vi "FPGATest.vi"() -> ()   [LabVIEW 2016]
uses:
  <vilib>/Platform/TimedLoop/XDataNode/timing_clust.ctl
  <vilib>/Platform/TimedLoop/XDataNode/nitl_modes.ctl
  <vilib>/Platform/TimedLoop/XDataNode/wakeup.ctl
  <userlib>/_NI SPI IP/FPGA/Controllers/Public/Transfer Settings.ctl
  <userlib>/_NI SPI IP/FPGA/Controllers/Public/Slave Transfer Settings.ctl
  <vilib>/rvi/Emulation/niFpgaSctlEmulationGetInTimedLoop.vi
  <vilib>/rvi/Emulation/niFpgaEmulationReportErrorSimple.vi
  <vilib>/rvi/Emulation/niFpgaGetClockAttributes.vi
  <vilib>/rvi/Emulation/niFpgaCriticalErrorInLSC.vi
  <vilib>/rvi/eio/common/nirviEmuTemplateMethod_errors.vi
  <vilib>/platform/TimedLoop/XDataNode/XDataNode.xnode
  <vilib>/eio/EIONode/EIONode.xnode
  <userlib>/_NI SPI IP/FPGA/Controllers/NI SPI IP FPGA.lvlib
  <vilib>/Platform/TimedLoop/XDataNode/XDNodeRunTimeDep.lvlib
panel:
  out "ready for input":bool
  in  "start strobe":bool
  in  "MOSI output enable done":bool=TRUE
  out "read data":u64 format="%.0x"
  out "read data valid":bool
  in  "data to write":u64 format="%.0x"
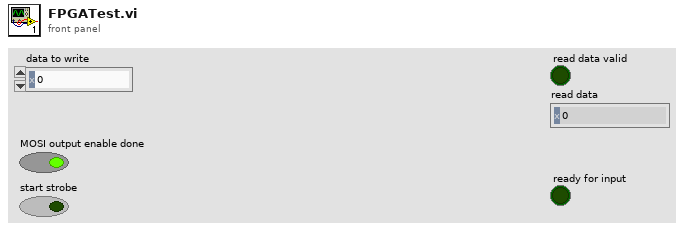
[diagram p1: front panel]
types:
  T1 = typedef "XDNodeRunTimeDep.lvlib/timing_clust.ctl" = cluster{"Expected End [f-1]":u64, "Actual End [f-1]":u64, "Finished Late? [f-1]":bool, "Expected End [i-1]":u64, "Actual End [i-1]":u64, "Finished Late? [i-1]":bool, "Expected Start [i]":u64, "Actual Start [i]":u64, "Expected Start [f]":u64, "Actual Start [f]":u64, "Source Name":string, "Structure Name":string, "Period":i64, "Deadline":i64, "Offset":i64, "Start":i64, "Priority":i32, "Timeout":i32, "Mode":T2, "Wakeup Reason":T3, "Error":errorcluster, "Source Type":string, "Secondary Source Type":string, "Global End Time":u64, "Global Start Time":u64, "Frame Duration":u64, "Iteration Duration":u64, "Assigned CPU":i32, "I/O Scan Engine Mode":u32}
  T2 = typedef "XDNodeRunTimeDep.lvlib/nitl_modes.ctl" = enum32{"No Change", "Process missed periods, maintain original phase", "Discard missed periods, maintain original phase", "Process missed periods, ignore original phase", "Discard missed periods, ignore original phase"}
  T3 = typedef "XDNodeRunTimeDep.lvlib/wakeup.ctl" = enum32{"Normal", "Aborted", "Asynchronous wakeup", "Timing source error", "Timed loop error", "Timeout"}
  T4 = typedef "NI SPI IP FPGA.lvlib/Transfer Settings.ctl" = cluster{"Divide Value":u8, "Transfer Length (bits)":u8, "CS Asserted Polarity":bool, "Clock Polarity (CPOL)":bool, "Clock Phase (CPHA)":bool, "Lengthen MISO Setup":bool, "Direction Change Bit":u8, "MOSI Starts as Output":bool, "Tristatable MOSI":bool}
  T5 = typedef "NI SPI IP FPGA.lvlib/Slave Transfer Settings.ctl" = cluster{"Transfer Length (bits)":u8, "CS Asserted Polarity":bool, "Clock Polarity (CPOL)":bool, "Clock Phase (CPHA)":bool}
  T6 = typedef "NI SPI IP FPGA.lvlib/Spi Master Outputs.ctl" = cluster{"Chip Select":bool, "Clock":bool, "MOSI":bool, "MOSI OE":bool}
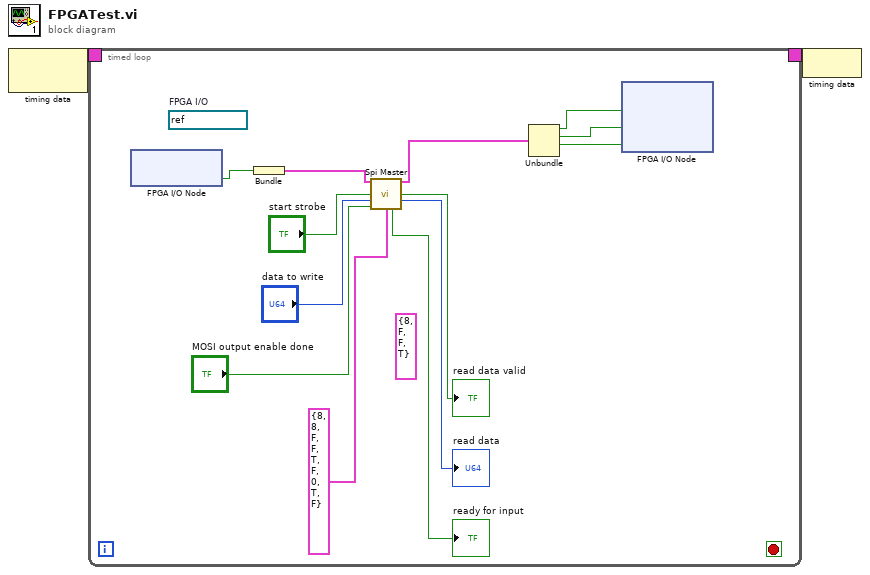
[diagram p0: block diagram]
diagram:
  n1 = node-c288() -> (w2:T1)  [unwired: 1 in]
  n2 = timed-loop {
    timing: w2 -> [_]
    timing-out: [_] -> w1
    stop <- _ stop-if-true
    (unwired) refnum<k21> "DIO/DIO1"  # FPGA I/O
    (unwired) T5 {"Transfer Length (bits)"=8, "CS Asserted Polarity"=FALSE, "Clock Polarity (CPOL)"=FALSE, "Clock Phase (CPHA)"=TRUE} ("transfer settings")
    n3 = xnode "FPGA I/O Node"() -> ("SPI MISO"=w7:bool)  [unwired: 1 in, 1 out]
    n4 = Bundle("SPI MISO"=w7) -> (w6:cluster{"SPI MISO":bool})  [unwired: 1 in]
    n5 = call <userlib>:"Spi Master.vi"("spi input"=w6, "start strobe"="start strobe", "data to write"="data to write", "MOSI output enable done"="MOSI output enable done", "spi transfer settings"=T4 {"Divide Value"=8, "Transfer Length (bits)"=8, "CS Asserted Polarity"=FALSE, "Clock Polarity (CPOL)"=FALSE, "Clock Phase (CPHA)"=TRUE, "Lengthen MISO Setup"=FALSE, "Direction Change Bit"=0, "MOSI Starts as Output"=TRUE, "Tristatable MOSI"=FALSE}) -> ("spi output"=w8:T6, "read data valid"=→"read data valid":bool, "read data"=→"read data":u64, "ready for input"=→"ready for input":bool)  [unwired: 7 in]
    n6 = Unbundle(w8) -> ("Chip Select"=w5:bool, "Clock"=w4:bool, "MOSI"=w3:bool)  [unwired: 1 out]
    n7 = xnode "FPGA I/O Node"("SPI CS0"=w5, "SPI CLK"=w4, "SPI MOSI"=w3) -> ()  [unwired: 3 in, 3 out]
  }
  n8 = node-c288(w1) -> ()
